vi "yearly breakdown query 2.vi"(7 "String 2":string, 8 "error in (no error)":errorcluster, 9 "?":i32, 10 "String":string, 11 "Refnum in":T1) -> (0 "error out":errorcluster, 1 "Count":i32, 2 "sum":dbl, 3 "Refnum out":T1)   [LabVIEW 2017]
uses:
  <vilib>/addons/database/Connection.llb/Conn ObjectReference.ctl
  <vilib>/addons/database/Connection.llb/Conn Execute.vi
  <vilib>/addons/database/Recordset.llb/Rec Fetch Recordset Data (R).vi
  <vilib>/addons/database/Recordset.llb/Rec Destroy - Connection.vi
  <vilib>/addons/database/NI_Database_API.lvlib
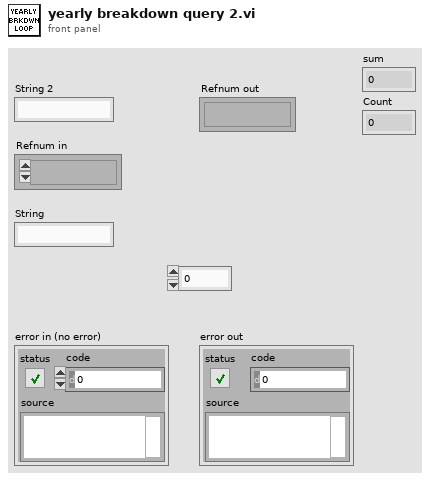
[diagram p1: front panel]
types:
  T1 = typedef "NI_Database_API.lvlib/Conn ObjectReference.ctl" = refnum<k1>
  T2 = typedef "NI_Database_API.lvlib/Rec ObjectReference.ctl" = refnum<k1>
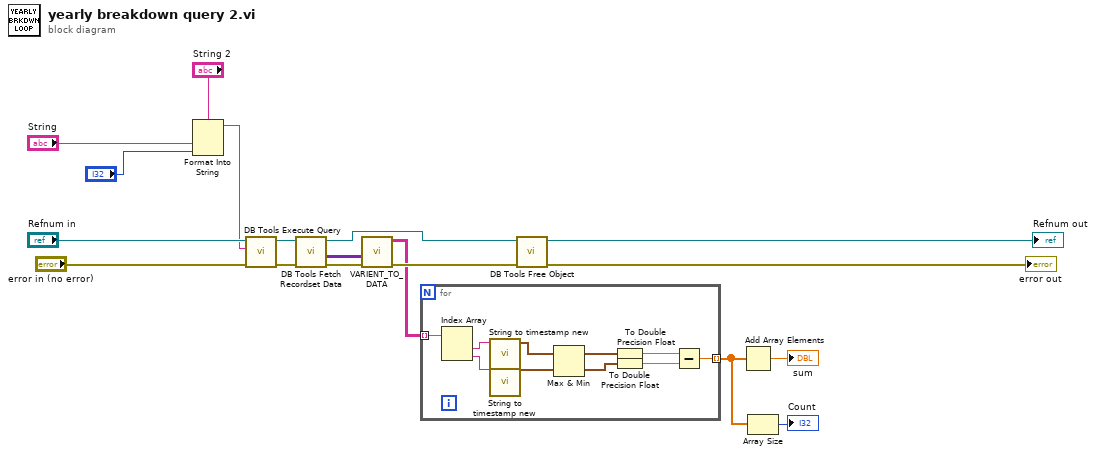
[diagram p0: block diagram]
diagram:
  n1 = Format Into String(format string="String 2", "String", "?") -> (resulting string=w6:string)  [unwired: 2 in, 1 out]
  n2 = call-poly <vilib>:"DB Tools Execute Query.vi"("error in (no error)"="error in (no error)", "SQL query"=w6, "connection reference"="Refnum in") -> ("error out"=w12:errorcluster, "recordset reference"=w10:T2)  [unwired: 5 in]
  n3 = call-poly <vilib>:"DB Tools Fetch Recordset Data.vi"("error in (no error)"=w12, "recordset reference"=w10) -> ("error out"=w11:errorcluster, "recordset data"=w7:variant[][], "recordset reference out"=w9:T2)  [unwired: 3 in]
  n4 = call "VARIENT_TO_DATA.vi"("data"=w7, "error in (no error)"=w11) -> ("Table"=w5:string[][], "error out"=w8:errorcluster)  [unwired: 7 in]
  n5 = for {
    tunnel: w5 -> [w20] mode=indexing
    tunnel: [w19] -> w2 mode=indexing
    n6 = Index Array(array=w20) -> (element #1=w22:string, element #2=w21:string)  [unwired: 2 in]
    n7 = call "String to timestamp new.vi"("String Timestamp"=w22) -> ("Timestamp"=w24:timestamp)  [unwired: 10 in]
    n8 = call "String to timestamp new.vi"("String Timestamp"=w21) -> ("Timestamp"=w23:timestamp)  [unwired: 10 in]
    n9 = Max & Min(x=w24, y=w23) -> (max(x,y)=w28:timestamp, min(x,y)=w27:timestamp)
    n10 = To Double Precision Float(number=w28) -> (double precision float=w26:dbl)
    n11 = To Double Precision Float(number=w27) -> (double precision float=w25:dbl)
    n12 = Subtract(x=w26, y=w25) -> (x-y=w19:dbl)
  }
  n13 = call-poly <vilib>:"DB Tools Free Object.vi"("error in (no error)"=w8, "recordset reference"=w9) -> ("error out"=→"error out":errorcluster, "connection reference"=→"Refnum out":T1)  [unwired: 8 in]
  n14 = Add Array Elements(numeric array=w2) -> (sum=→"sum":dbl)
  n15 = Array Size(array=w2) -> (size(s)=→"Count":i32)
